vi "抓取天气查询.vi"(1 "城市（市，县）":string) -> (0 "当前天气":string)   [LabVIEW 2016]
uses:
  <vilib>/regexp/Match Regular Expression.xnode
  <vilib>/httpClient/LabVIEWHTTPClient.lvlib
panel:
  out "error out":errorcluster caption="错误输出"
  out "查询结果":string
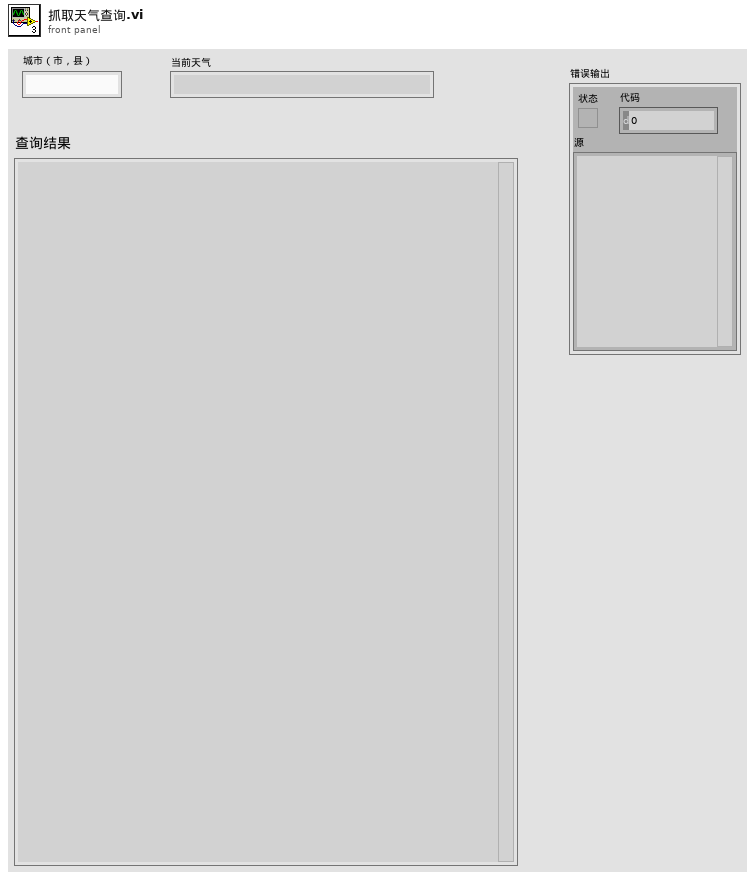
[diagram p1: front panel]
types:
  T1 = typedef "LabVIEWHTTPClient.lvlib/ClientHandle.ctl" = refnum<k1>
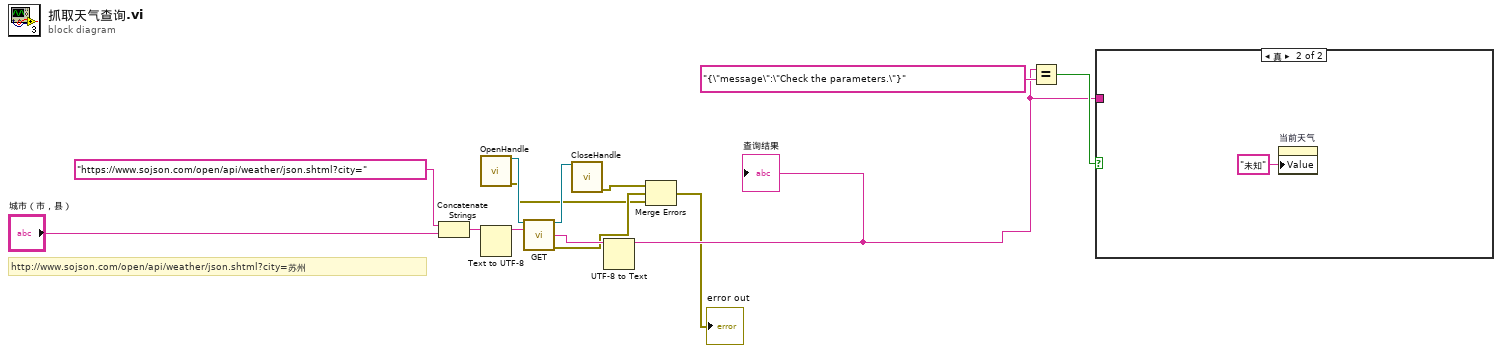
[diagram p0: block diagram]
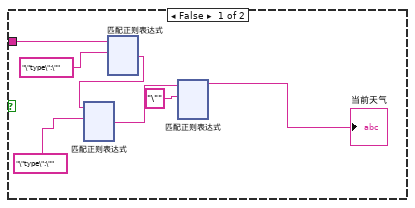
[diagram p2: hidden frame]
diagram:
  # "http://www.sojson.com/open/api/weather/json.shtml?city=苏州"
  n1 = Concatenate Strings("https://www.sojson.com/open/api/weather/json.shtml?city=" ("字符串"), "城市（市，县）") -> (w8:string)
  n2 = call <vilib>:"OpenHandle.vi"() -> ("client handle out"=w13:T1, "error out"=w2:errorcluster)  [unwired: 14 in]
  n3 = Text to UTF-8(11:w8) -> (3:w10:string)  [unwired: 2 in, 1 out]
  n4 = call <vilib>:"GET.vi"("client handle"=w13, "url"=w10) -> ("client handle out"=w12:T1, "body"=w11:string, "error out"=w3:errorcluster)  [unwired: 10 in, 1 out]
  n5 = call <vilib>:"CloseHandle.vi"("client handle"=w12) -> ("error out"=w4:errorcluster)  [unwired: 14 in]
  n6 = UTF-8 to Text(11:w11) -> (3:w5:string)  [unwired: 2 in, 1 out]
  "查询结果" <- w5
  n7 = Merge Errors(w4, w3, w2) -> (→"error out":errorcluster)
  n8 = Equal?(x=w5, y="{\"message\":\"Check the parameters.\"}") -> (x = y?=w6:bool)
  n9 = case shown="真" w6 {
    tunnel: w5 -> [w15 _]
    frame False {
      n10 = xnode "匹配正则表达式"("输入字符串"=w15, "正则表达式"="\"type\":\"") -> ("匹配之后"=w21:string)  [unwired: 4 in, 4 out]
      n11 = xnode "匹配正则表达式"("输入字符串"=w21, "正则表达式"="\"type\":\"") -> ("匹配之后"=w18:string)  [unwired: 4 in, 4 out]
      n12 = xnode "匹配正则表达式"("输入字符串"=w18, "正则表达式"="\"") -> ("匹配之前"=→"当前天气":string)  [unwired: 4 in, 4 out]
    }
    frame True {
      n13 = property on="当前天气" class="Str"("Value"="未知" ("当前天气")) -> ()  [unwired: 2 in, 2 out]
    }
  }
